vi "ejercicio 2.vi"() -> ()   [LabVIEW 2017]
panel:
  out "suma columnas":i64[](array[numeric])
  out "Min":i64
  out "Max":i64
  out "Promedio":dbl
  out "Arreglo":i64[][](array[numeric])
  # "Ejercicio 2\nEscriba un programa que ponga numeros aleatorios menores a 100 en un arreglo bidimensional\nde 5x4. Se pide:\nCalcular promedio de todos los numeros\nMostrar el valor maximo y minimo"
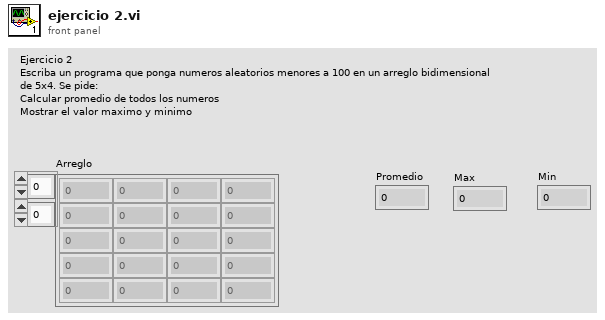
[diagram p1: front panel]
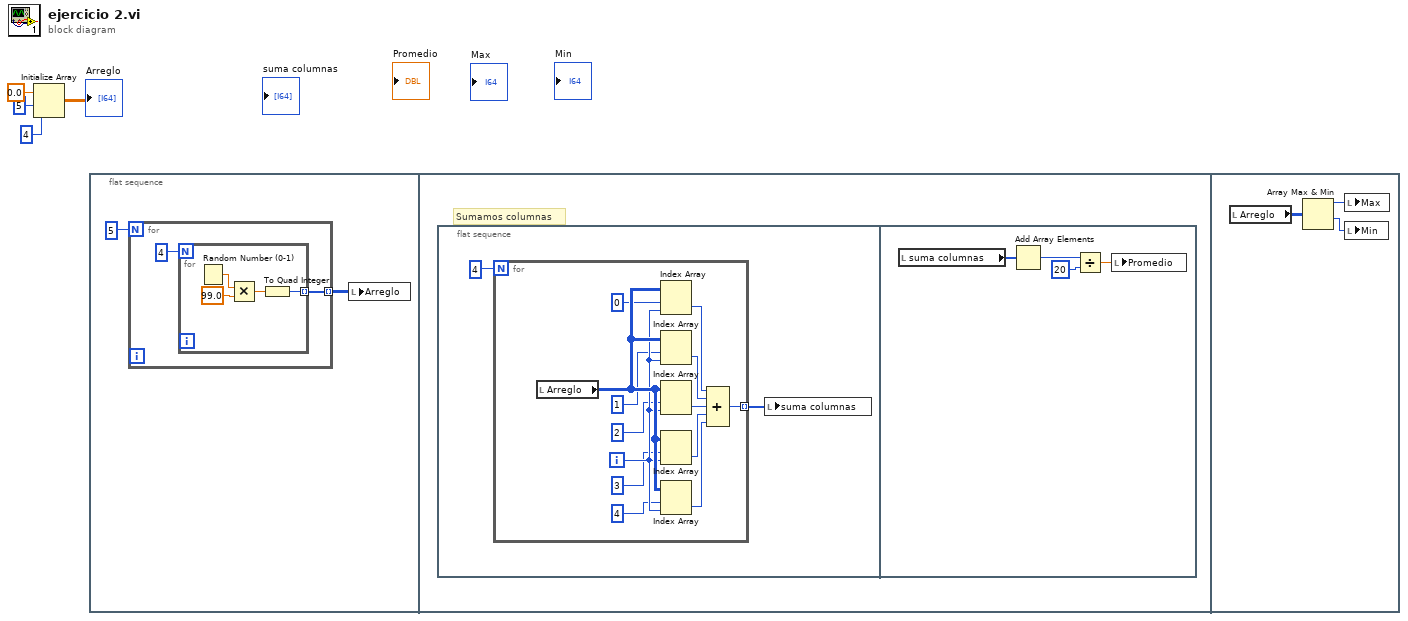
[diagram p0: block diagram]
diagram:
  n1 = Initialize Array(0.0 ("element"), 5 ("dimension size"), 4 ("dimension size")) -> (→"Arreglo":dbl[][])
  n2 = flat-sequence {
    frame #0 {
      n3 = for {
        N: 5 -> [_]
        tunnel: [w7] -> w5 mode=indexing
        n4 = for {
          N: 4 -> [_]
          tunnel: [w9] -> w7 mode=indexing
          n5 = Random Number (0-1)() -> (number: 0 to 1=w12:dbl)
          n6 = Multiply(x=w12, y=99.0) -> (x*y=w10:dbl)
          n7 = To Quad Integer(1:w10) -> (0:w9:i64)
        }
      }
      n8 = local write "Arreglo"(w5) -> ()
    }
    frame #1 {
      # "Sumamos columnas"
      n9 = flat-sequence {
        frame #0 {
          n10 = for {
            N: 4 -> [_]
            tunnel: [w15] -> w13 mode=indexing
            i -> [w26]
            n11 = local read "Arreglo"() -> (w27:i64[][])
            n12 = Index Array(array=w27, index (row)=0 ("disabled index (row)"), index (col)=w26) -> (element=w20:i64)
            n13 = Index Array(array=w27, index (row)=1 ("disabled index (row)"), index (col)=w26) -> (element=w19:i64)
            n14 = Index Array(array=w27, index (row)=2 ("disabled index (row)"), index (col)=w26) -> (element=w18:i64)
            n15 = Index Array(array=w27, index (row)=3 ("disabled index (row)"), index (col)=w26) -> (element=w17:i64)
            n16 = Index Array(array=w27, index (row)=4 ("disabled index (row)"), index (col)=w26) -> (element=w16:i64)
            n17 = Compound Arithmetic op=ADD(w20, w19, w18, w17, w16) -> (w15:i64)
          }
          n18 = local write "suma columnas"(w13) -> ()
        }
        frame #1 {
          n19 = local read "suma columnas"() -> (w31:i64[])
          n20 = Add Array Elements(numeric array=w31) -> (sum=w30:i64)
          n21 = Divide(x=w30, y=i64 20) -> (x/y=w28:dbl)
          n22 = local write "Promedio"(w28) -> ()
        }
      }
    }
    frame #2 {
      n23 = local read "Arreglo"() -> (w34:i64[][])
      n24 = Array Max & Min(array=w34) -> (max value=w33:i64, min value=w32:i64)  [unwired: 2 out]
      n25 = local write "Max"(w33) -> ()
      n26 = local write "Min"(w32) -> ()
    }
  }
